vi "Global_TestConf.vi"() -> ()   [LabVIEW 2020]
panel:
  out "Test Type (OUTPUT)":string
  out "CAPACITANCE TEST?":bool
  in  "IGBT : Test Type":string[](array[string])
  in  "Transistor : Test Type":string[](array[string])
  in  "MOSFET : Test Type":string[](array[string])
  out "Test_Conf : error out":errorcluster
  in  "Test_Conf : error in":errorcluster
  out "Fixture File Name":string
  in  "Confirm Configuration":bool
  in  "Test Signal Level":string(combo)
  out "Device Type (OUTPUT)":string
  in  "Test Fixtures":u16(ring) items=["Diode & Bipolar Capacitance Adapter Box 1, CAP 1, BCE", "Diode & Bipolar Capacitance Adapter Box 1, CAP 2, BCE", "Diode & Bipolar Capacitance Adapter Box 1, CAP 2, ECB", "Diode & Bipolar Capacitance Adapter Box 1, CAP 5, BCE", "Diode & Bipolar Capacitance Adapter Box 1, CAP 5, ECB", "Diode & Bipolar Capacitance Adapter Box 1, CAP 6, BCE", "DIODE & BIPOLAR Multi-pin Capacitance fixture"]
  out "LowCapMode?":bool
  in  "Category":T1(ring)
  in  "Device Types":u16(ring) items=["Diode (Rectifier & Zener)", "Transistor", "BRT", "MOSFET", "JFET", "SSOVP", "SIDAC", "Bidirectional Zener", "SCR or TRIAC", "Darlington Transistor", "MicroIntegration", "MOSFET with Gate Resistor", "IGBT", "IGBT with Gate Resistor", "Other"]
  out "Test Fixture (OUTPUT)":string
  out "Test Types":string
  # "Category"
  # "Normal Mode is only for : \n\nDiode (Rectifier & Zener)\nBidirectional Zener\nMicroIntegration\nOther"
  # "Diode :\n----------------------\n0) Diode\n7) Bidirectional Zener"
  # "TRUE : Normal Mode\nFALSE : Hi-RES"
  # "Thyristor :\n---------------------\n5) SSOVP\n6) SIDAC\n8) SRC or TRIAC\n10) MicroIntegration\n14) Other"
  # "Transistor :\n------------------------\n1) Transistor\n2) BRT\n9) Darlington Transistor"
  # "MOSFET :\n-------------------------------\n3) MOSFET\n4) JFET\n11) MOSFET with Gate Resistor"
  # "Checking"
  # "If RG, it will be false"
  # "IGBT :\n----------------------------\n12) IGBT\n13) IGBT with Gate Resistor"
  # "--------------------------------------------------------------------------------------------------------------------------------OLD----------------------------------------------------------------------------------------------------"
  # "IGBT"
  # "MOSFET"
  # "Test Fixture"
  # "Test Fixture"
  # "Diode & Bipolar Capacitance Adapter Box 1, CAP 4\nRG TEST FIXTURE 4284A 4285A E4980A \nBLACK SAP :  CRD / CRSS FIXTURE (VDS is variable, VGS=0V)\nBLACK SAP :  COD / COSS FIXTURE\t(VDS is variable, VGS=0V)\nBLACK SAP :  CID / CISS FIXTURE\t(VDS is variable, VGS=0V)\nRED SAP :  CRD / CRSS FIXTURE\t(VGS is variable, VDS=0V)\nRED SAP :  CID / CISS FIXTURE\t(VGS is variable, VDS=0V)\nMOSFET Multi-pin COSS Capacitance fixture (VDS is variable, VGS=0V)\nMOSFET Multi-pin CISS Capacitance fixture (VDS is variable, VGS=0V)\nMOSFET Multi-pin CRSS Capacitance fixture (VDS is variable, VGS=0V)"
  # "Diode & Bipolar Capacitance Adapter Box 1, CAP 4\nRG TEST FIXTURE 4284A 4285A E4980A \nBLACK SAP :  CRD / CRSS FIXTURE (VDS is variable, VGS=0V)\nBLACK SAP :  COD / COSS FIXTURE\t(VDS is variable, VGS=0V)\nBLACK SAP :  CID / CISS FIXTURE\t(VDS is variable, VGS=0V)\nRED SAP :  CRD / CRSS FIXTURE\t(VGS is variable, VDS=0V)\nRED SAP :  CID / CISS FIXTURE\t(VGS is variable, VDS=0V)\nMOSFET Multi-pin COSS Capacitance fixture (VDS is variable, VGS=0V)\nMOSFET Multi-pin CISS Capacitance fixture (VDS is variable, VGS=0V)\nMOSFET Multi-pin CRSS Capacitance fixture (VDS is variable, VGS=0V)"
  # "Test Type"
  # "Test Type"
  # "CISS: VDS is variable, VGS=0V BLACK Jacks\nCOSS: VDS is variable, VGS=0V BLACK Jacks\nCRSS: VDS is variable, VGS=0V BLACK Jacks\nCISS: VDS is variable, VGS=0V RED Jacks\nCOSS: VDS is variable, VGS=0V RED Jacks\nCRSS: VDS is variable, VGS=0V RED Jacks\n\nRG\nSpecial"
  # "CIES: VDS is variable, VGS=0V BLACK Jacks\nCOES: VDS is variable, VGS=0V BLACK Jacks\nCRES: VDS is variable, VGS=0V BLACK Jacks\nCIES: VGS is variable, VDS=0V RED Jacks\nCOES: VGS is variable, VDS=0V RED Jacks\nCRES: VGS is variable, VDS=0V RED Jacks\n\nRG\nSpecial"
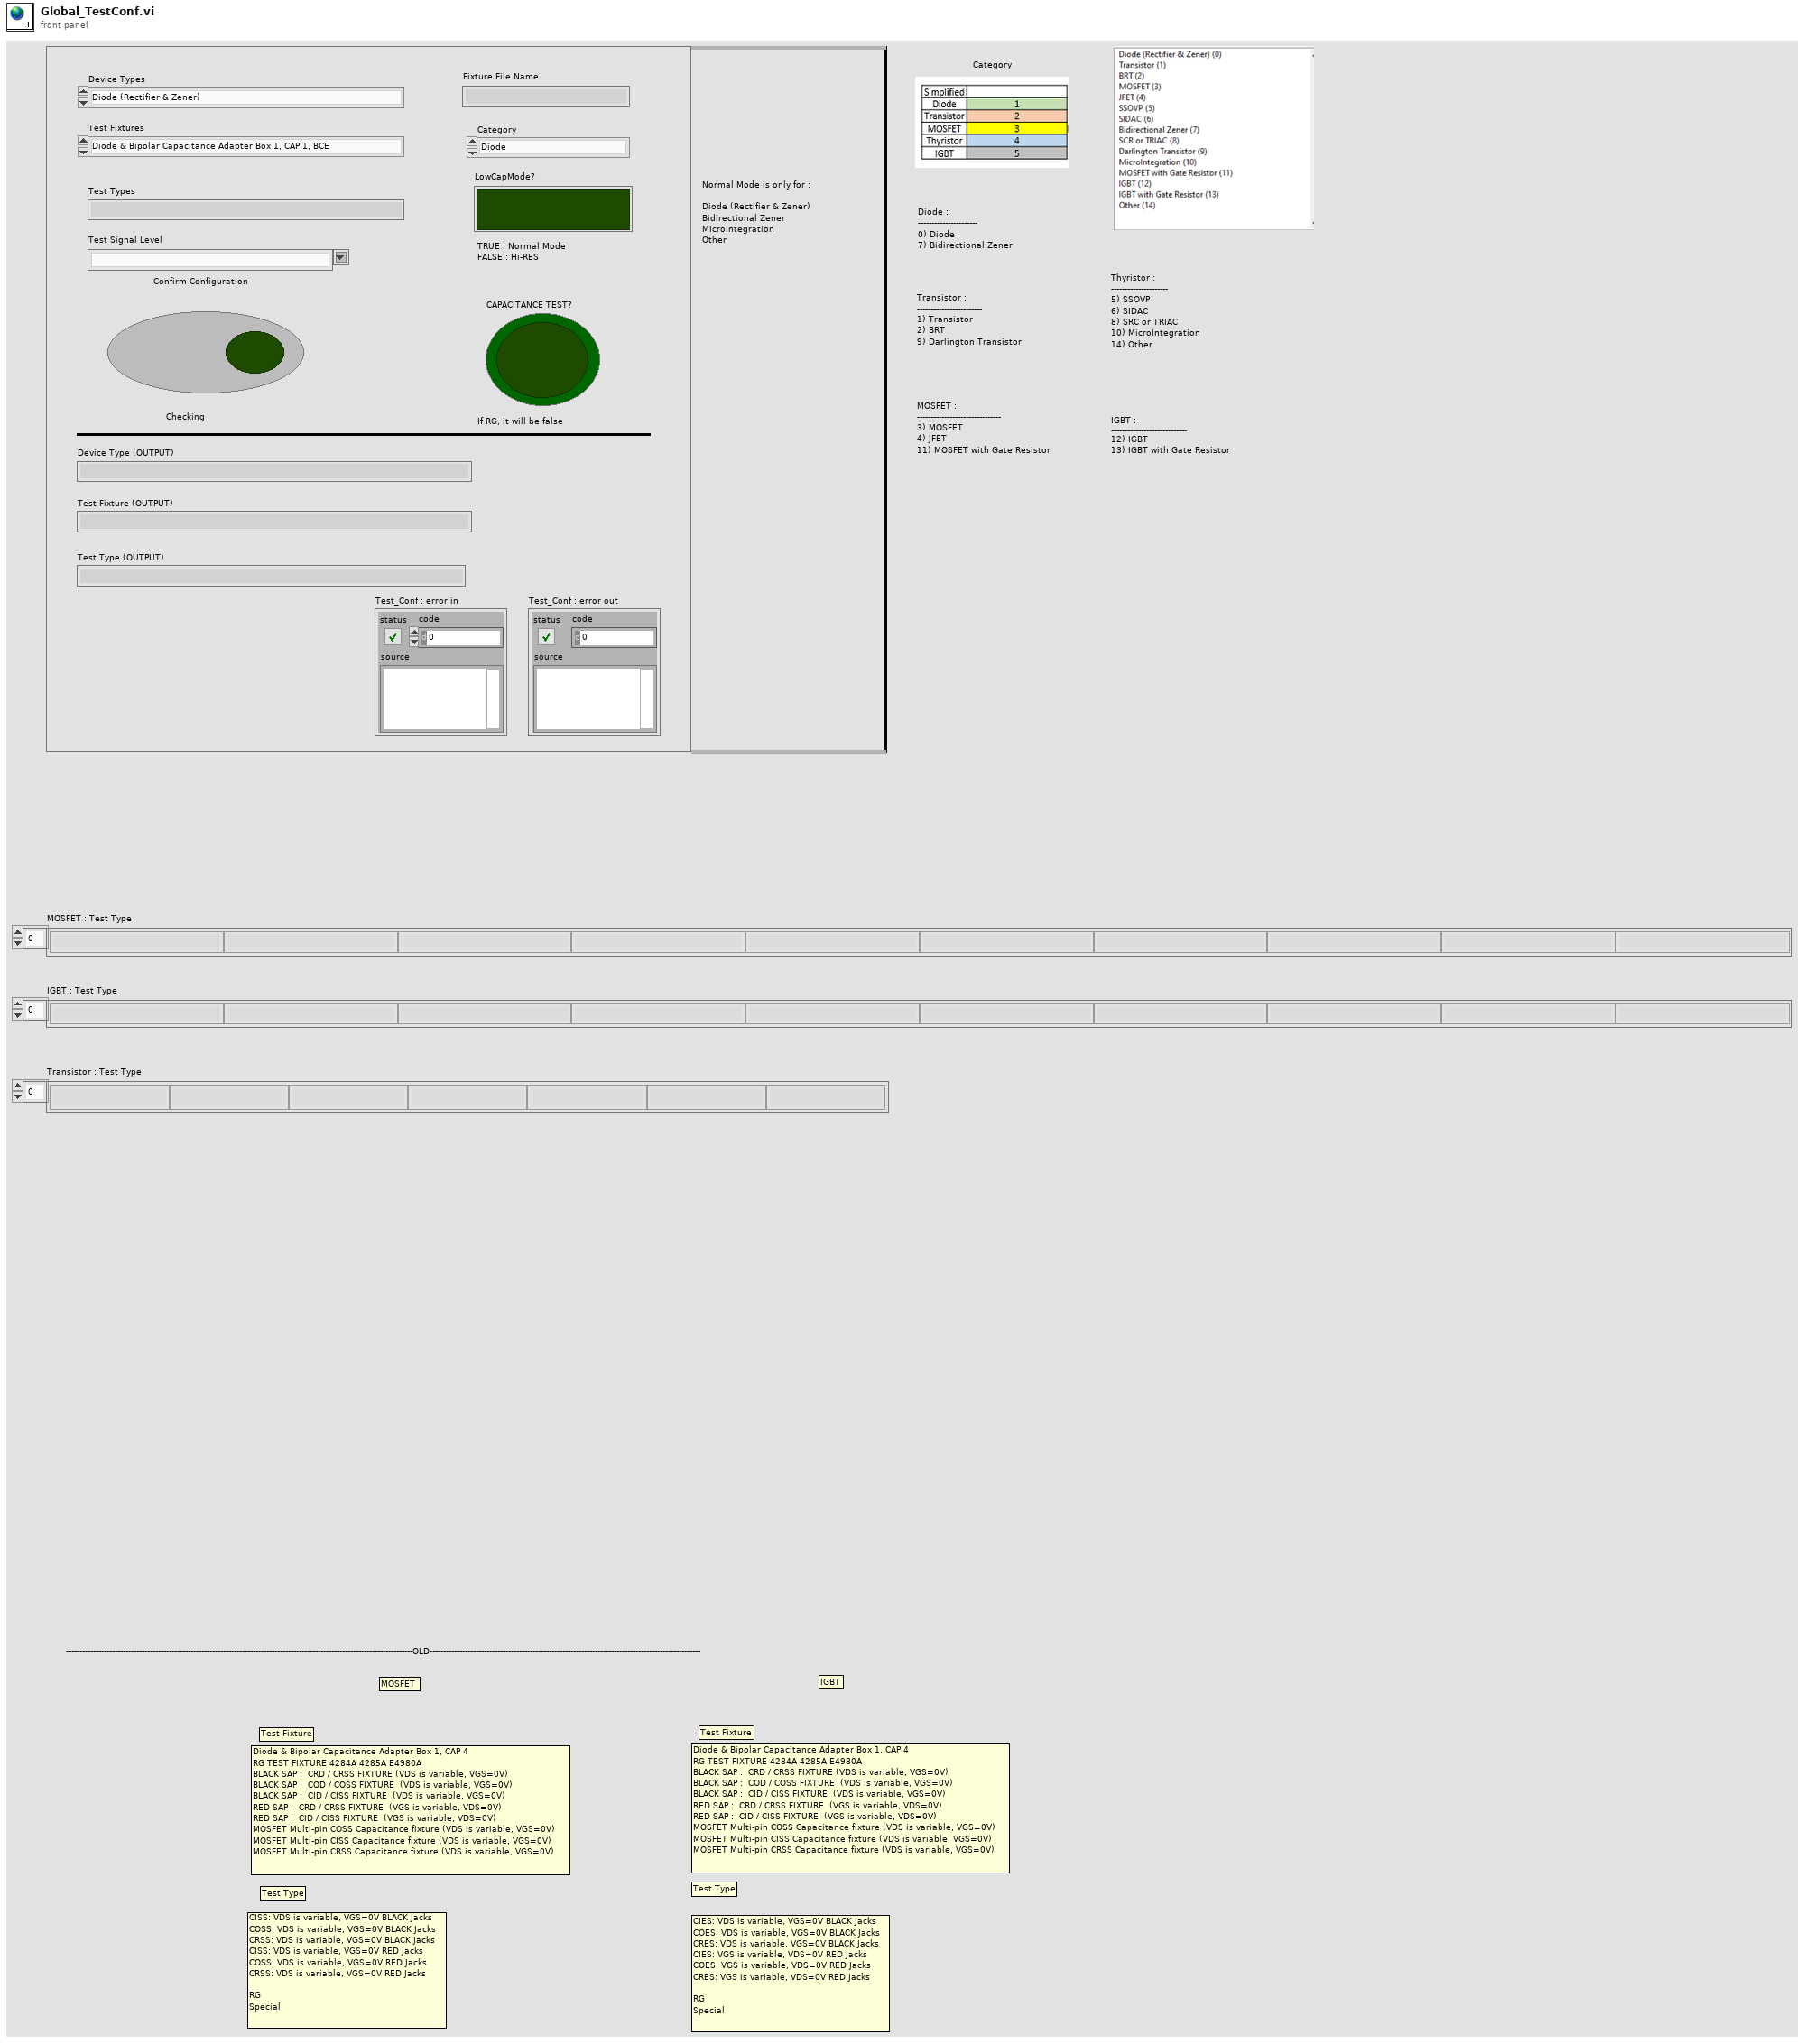
[diagram p1: front panel]
types:
  T1 = enum16{"Diode", "Transistor", "MOSFET", "Thyristor", "IGBT"}
diagram:
